vi "CDMA_RxRFloopback.vi"(6 "pcip":string, 7 "xsrpip":string, 8 "error in (no error)":errorcluster caption="错误输入（无错误）", 9 "system_type":dbl, 10 "tx_data":dbl[](array[numeric]), 11 "Path In":path) -> (0 "error out":errorcluster caption="错误输出", 2 "rxData":cdb[](array[numeric]), 3 "Path Out":path)   [LabVIEW 2015]
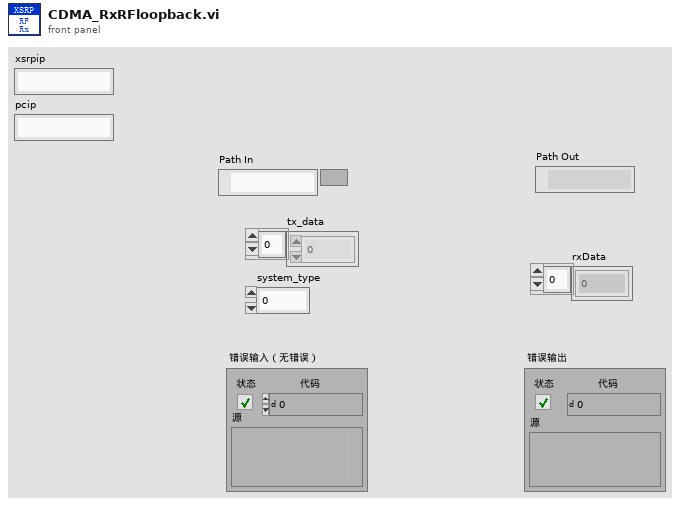
[diagram p1: front panel]
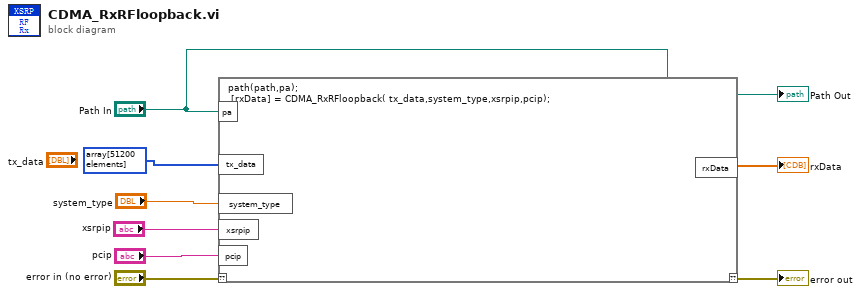
[diagram p0: block diagram]
diagram:
  n1 = script code="path(path,pa);\n [rxData] = CDMA_RxRFloopback( tx_data,system_type,xsrpip,pcip);"("??"="error in (no error)", "pa"="Path In", "tx_data"=i32[] array[51200 elements], "system_type"="system_type", "xsrpip"="xsrpip", "pcip"="pcip") -> ("??"=→"error out":errorcluster, "rxData"=→"rxData":cdb[])
  "Path Out" <- "Path In"
